vi "Quick Usb Async Wait.vi"(7 "immediate":u8, 8 "error in (no error)":errorcluster, 9 "transaction":u8, 10 "bytecount":u32, 11 "hDevice":u32) -> (0 "error out":errorcluster, 1 "function return":i32, 2 "bytecount out":u32, 3 "hDevice out":u32)   [LabVIEW 2011, in "QuickUSB.lvlib"]
doc: "QUSBLIB QRETURN QuickUsbAsyncWait(\n QHANDLE hDevice, \n PQULONG bytecount,\n QBYTE transaction,\n QBYTE immediate\n);"
uses:
  QuickUSB.lvlib
  QuickUSB.dll
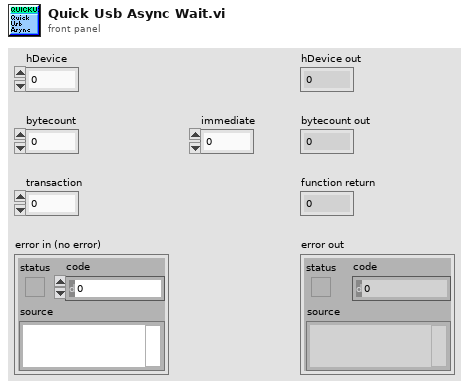
[diagram p1: front panel]
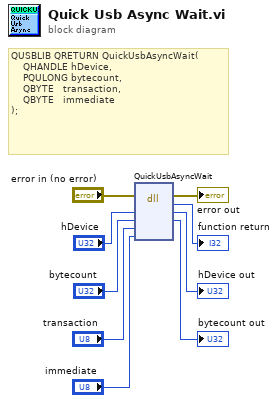
[diagram p0: block diagram]
diagram:
  # "QUSBLIB QRETURN QuickUsbAsyncWait(\n    QHANDLE hDevice, \n    PQULONG bytecount,\n    QBYTE   transaction,\n    QBYTE   immediate\n);"
  n1 = dll-call lib="C:/QuickUSB/QuickUSB.*" fn="QuickUsbAsyncWait"(error in="error in (no error)", "hDevice"="hDevice", "bytecount"="bytecount", "transaction"="transaction", "immediate"="immediate") -> (error out=→"error out":errorcluster, →"function return":i32, "hDevice"=→"hDevice out":u32, "bytecount"=→"bytecount out":u32)  [unwired: 4 in, 1 out]
